vi "Read connectionTimeout.vi"(8 "error in (no error)":errorcluster, 11 "deviceHeartbeat in":refnum<class "deviceHeartbeat.lvclass">) -> (0 "error out":errorcluster, 2 "connected":bool, 3 "deviceHeartbeat out":refnum<class "deviceHeartbeat.lvclass">)   [LabVIEW 2016, in "deviceHeartbeat.lvclass"]
uses:
  deviceHeartbeat.lvclass
  deviceHeartbeat.lvclass/deviceHeartbeat.ctl
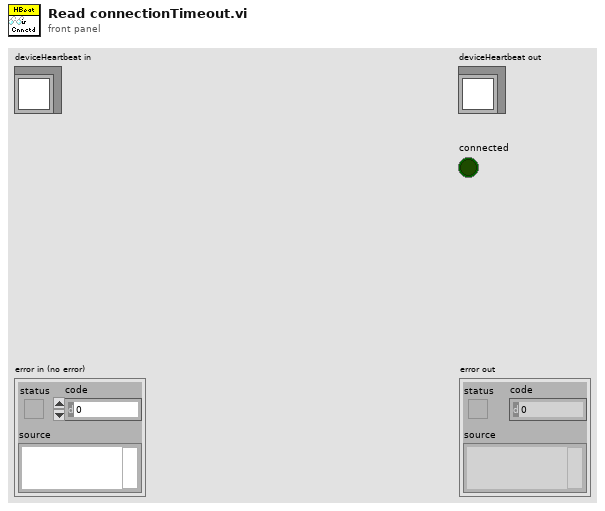
[diagram p1: front panel]
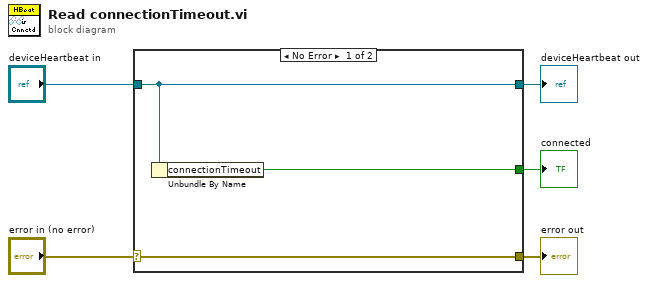
[diagram p0: block diagram]
diagram:
  n1 = case shown="No Error" "error in (no error)" {
    selector: "error in (no error)" -> [w8 w9]
    tunnel: [w8 w9] -> w4
    tunnel: [w7 w10] -> w2
    tunnel: "deviceHeartbeat in" -> [w7 w10]
    tunnel: [w6 _] -> w1
    frame No Error {
      n2 = Unbundle By Name(w7) -> ("connectionTimeout"=w6:bool)
    }
    frame Error {
    }
  }
  "error out" <- w4
  "deviceHeartbeat out" <- w2
  "connected" <- w1
